vi "Event.xio.vi"(6 "Error in":errorcluster caption="错误常量", 7 "标志事件":string, 9 "事件组":string[](array[string])) -> (0 "Error out":errorcluster caption="错误常量", 1 "？":bool, 2 "下一事件":string, 3 "下一事件组":string[](array[string]), 4 "上一事件":string)   [LabVIEW 2018]
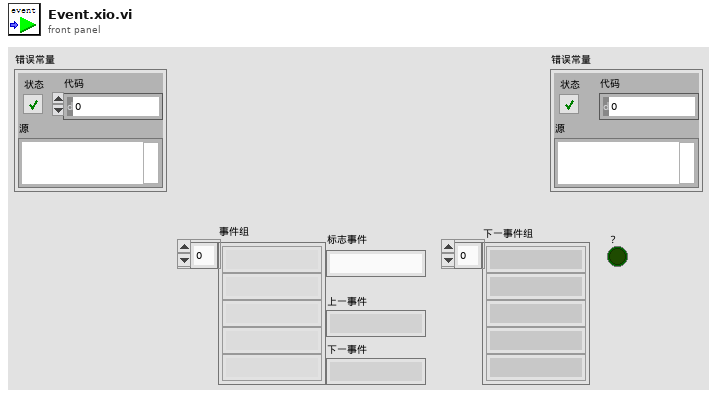
[diagram p1: front panel]
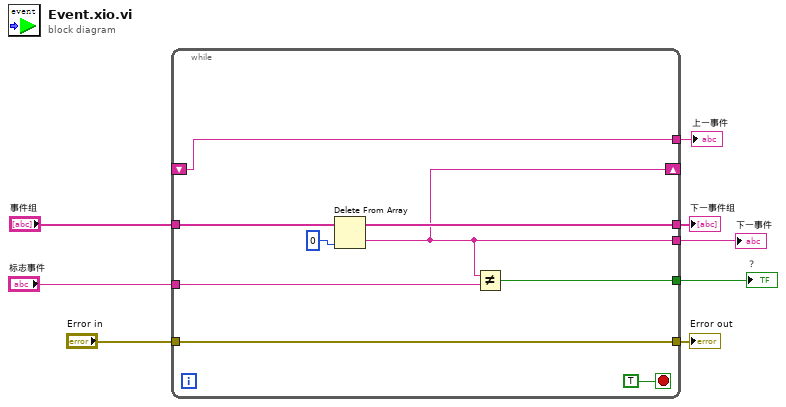
[diagram p0: block diagram]
diagram:
  n1 = while {
    tunnel: "标志事件" -> [w14]
    tunnel: [w13] -> w6
    tunnel: [w11] -> w4
    tunnel: "事件组" -> [w17]
    tunnel: [w12] -> w5
    shift-right: [w11] -> _
    shift-left: _ -> [w10]
    tunnel: [w10] -> w3
    tunnel: [w9] -> w1
    tunnel: "Error in" -> [w9]
    stop <- TRUE stop-if-true
    n2 = Delete From Array(array=w17, index=0 ("索引")) -> (deleted portion=w11:string, array with subset deleted=w12:string[])  [unwired: 1 in]
    n3 = Not Equal?(x=w11, y=w14) -> (x != y?=w13:bool)
  }
  "？" <- w6
  "下一事件组" <- w5
  "下一事件" <- w4
  "上一事件" <- w3
  "Error out" <- w1
